vi "App_Training Mode.vi"() -> ()   [LabVIEW 2015, in "Application 1.lvlib"]
uses:
  Application 1.lvlib
  Data Def/App_User Event Data.ctl
  Data Def/App_Subpanel Name.ctl
  Data Def/App_Tips Data.ctl
panel:
  in  "Action":bool
  out "Process":i32(slide) scale=0.0..10.0
  in  "Training Times":i32=10 caption="Numeric" min=1 max=1000 format="%.0f "
  out "Electrocardiography":waveform(dbl)(graph) caption="Waveform Graph"
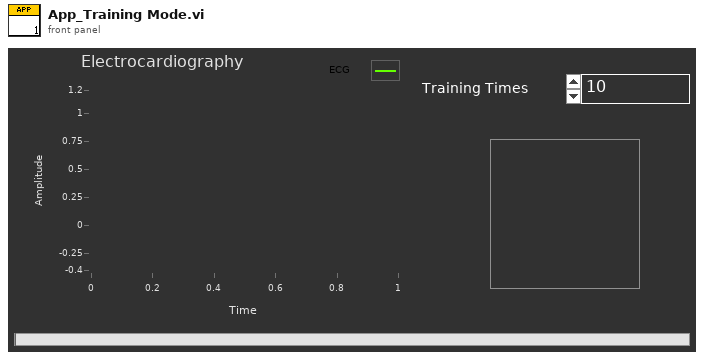
[diagram p1: front panel]
types:
  T1 = typedef "Application 1.lvlib/App_Subpanel Name.ctl" = enum16{"Main", "Menu", "User Registering", "User Setting", "Monitor", "Traning Mode", "Query Data", "Connect Setting"}
  T2 = typedef "Application 1.lvlib/App_User Event Data.ctl" = cluster{"Command":string, "Data":variant}
  T3 = typedef "Application 1.lvlib/App_Tips Data.ctl" = cluster{"Tips":string, "BG Color":u32}
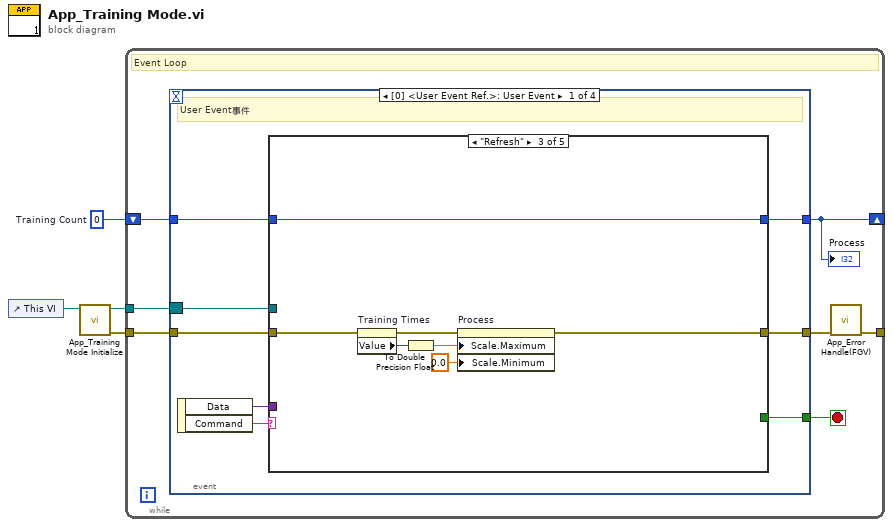
[diagram p0: block diagram]
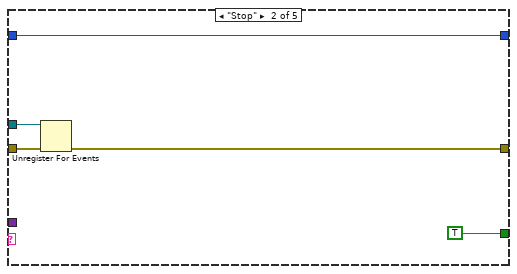
[diagram p3: hidden frame]
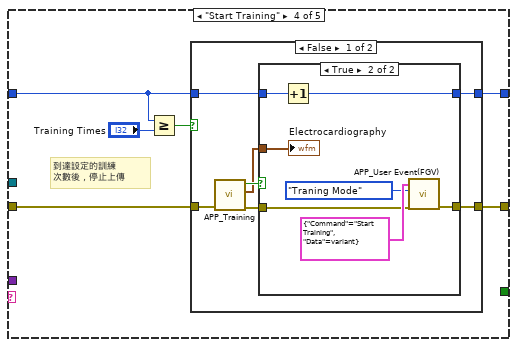
[diagram p4: hidden frame]
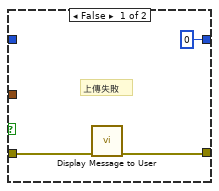
[diagram p5: hidden frame]
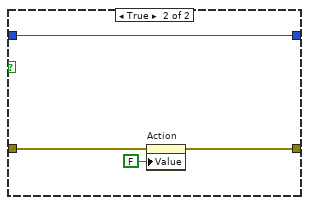
[diagram p6: hidden frame]
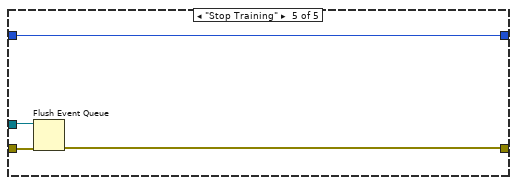
[diagram p7: hidden frame]
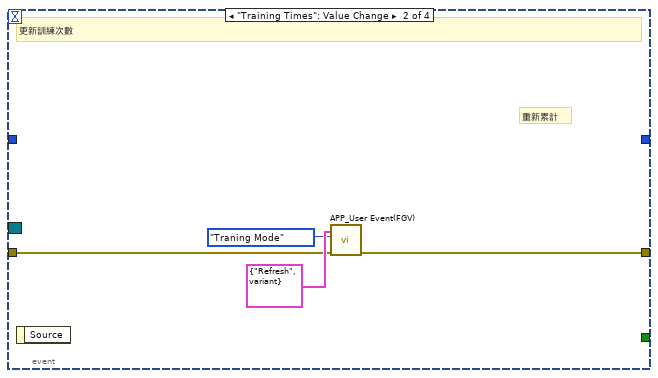
[diagram p8: hidden frame]
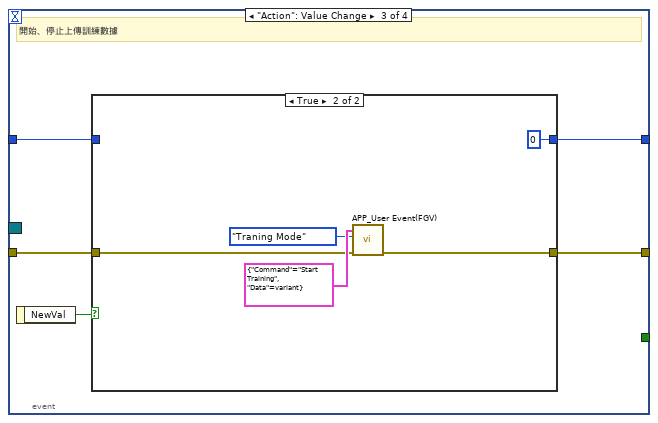
[diagram p9: hidden frame]
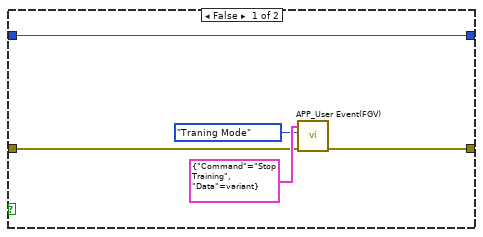
[diagram p10: hidden frame]
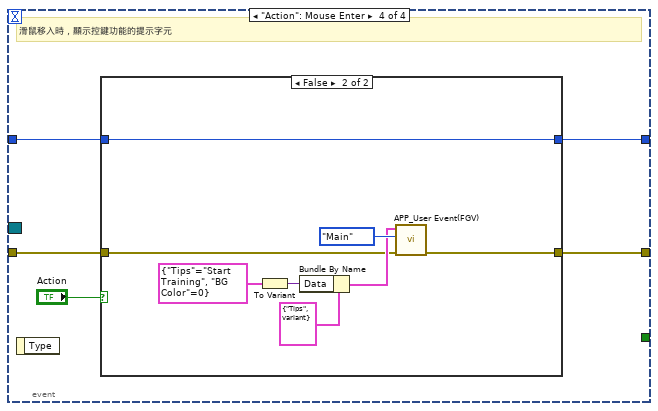
[diagram p11: hidden frame]
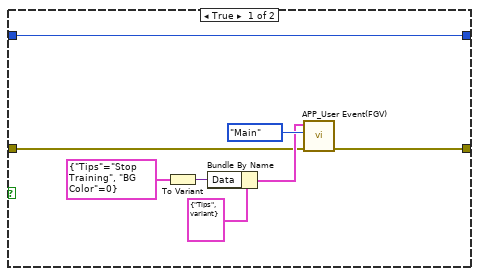
[diagram p12: hidden frame]
diagram:
  w1 = 0  # Training Count
  n1 = control-ref of="This VI"() -> (w4:refnum<vi>)
  n2 = call "App_Training Mode Initialize.vi"("VI Reference"=w4) -> ("error out"=w3:errorcluster, "Event Registration Refnum"=w2:refnum<event-registration>)  [unwired: 9 in]
  n3 = while {
    tunnel: w3 -> [w11]
    tunnel: w2 -> [w10]
    tunnel: [w8] -> _
    shift-right: [w5] -> _
    shift-left: w1 -> [w6]
    stop <- w7 stop-if-true
    # "Event Loop"
    n4 = event shown="[0] <User Event Ref.>: User Event" {
      selector: w10 -> [w15 _ _ _]
      dyn-events: _ -> [_ _ _ _]
      timeout: _ -> [_ _ _ _]
      tunnel: w11 -> [w17 w66 w73 w87]
      tunnel: [w16 w65 w72 w86] -> w9
      tunnel: [w14 _ _ _] -> w7
      tunnel: w6 -> [w13 _ w71 w85]
      tunnel: [w12 _ w70 w84] -> w5
      event User Event {
        # "User Event事件"
        n5 = event-data() -> ("Data"=w18:variant, "Command"=w19:string)  [unwired: 1 in]
        n6 = case shown="\"Refresh\"" w19 {
          tunnel: w18 -> [_ _ _ _ _]
          tunnel: w17 -> [w21 w26 w33 w34 w64]
          tunnel: [w21 w24 w28 w39 w62] -> w16
          tunnel: w15 -> [_ w25 _ _ w63]
          tunnel: [_ TRUE _ _ _] -> w14
          tunnel: w13 -> [w20 w22 w27 w36 w61]
          tunnel: [w20 w22 w27 w38 w61] -> w12
          frame Default {
          }
          frame "Stop" {
            n7 = Unregister For Events(event registration refnum=w25, error in=w26) -> (error out=w24:errorcluster)
          }
          frame "Refresh" {
            n8 = property on="Training Times" class="DigNum (strict)"(error in=w33) -> (error out=w31:errorcluster, "Value"=w32:i32)  [unwired: 1 in, 1 out]
            n9 = To Double Precision Float(number=w32) -> (double precision float=w30:dbl)
            n10 = property on="Process" class="Slide (strict)"(error in=w31, "Scale.Maximum"=w30, "Scale.Minimum"=0.0 ("Scale.Range:Minimum")) -> (error out=w28:errorcluster)  [unwired: 1 in, 1 out]
          }
          frame "Start Training" {
            # "到達設定的訓練\n次數後，停止上傳"
            n11 = Greater Or Equal?(x=w36, y="Training Times") -> (x >= y?=w35:bool)
            n12 = case shown="False" w35 {
              tunnel: w34 -> [w45 w59]
              tunnel: [w46 w57] -> w39
              tunnel: w36 -> [w42 w60]
              tunnel: [w41 w60] -> w38
              frame False {
                n13 = call "APP_Training.vi"("error in"=w45) -> ("error out"=w44:errorcluster, "Data"=w40:waveform(dbl), "OK?"=w43:bool)  [unwired: 8 in]
                n14 = case shown="True" w43 {
                  tunnel: [w47 w54] -> w46
                  tunnel: w44 -> [w48 w53]
                  tunnel: w42 -> [_ w52]
                  tunnel: [0 w51] -> w41
                  tunnel: w40 -> [_ w50]
                  frame False {
                    # "上傳失敗"
                    n15 = call "Display Message to User"("error in (no error)"=w48) -> ("error out"=w47:errorcluster)  [unwired: 9 in, 1 out]
                  }
                  frame True {
                    n16 = Increment(x=w52) -> (x+1=w51:i32)
                    n17 = call "APP_User Event(FGV).vi"("error in"=w53, "Subpanel Name"=App_Subpanel_Name."Traning Mode", "User Event Data"=T2 {"Command"="Start Training", "Data"=variant}) -> ("error out"=w54:errorcluster)  [unwired: 7 in, 1 out]
                    "Electrocardiography" <- w50
                  }
                }
              }
              frame True {
                n18 = property on="Action" class="Bool (strict)"(error in=w59, "Value"=FALSE ("Action")) -> (error out=w57:errorcluster)  [unwired: 1 in, 1 out]
              }
            }
          }
          frame "Stop Training" {
            n19 = Flush Event Queue(0:w63, 3:w64) -> (11:w62:errorcluster)  [unwired: 4 in, 2 out]
          }
        }
      }
      event "Training Times": Value Change {
        # "重新累計"
        # "更新訓練次數"
        n20 = event-data() -> ()  [unwired: 1 in, 1 out]
        n21 = call "APP_User Event(FGV).vi"("error in"=w66, "Subpanel Name"=App_Subpanel_Name."Traning Mode", "User Event Data"=T2 {"Command"="Refresh", "Data"=variant}) -> ("error out"=w65:errorcluster)  [unwired: 7 in, 1 out]
      }
      event "Action": Value Change {
        # "開始、停止上傳訓練數據"
        n22 = event-data() -> ("NewVal"=w69:bool)  [unwired: 1 in]
        n23 = case shown="True" w69 {
          tunnel: w73 -> [w76 w81]
          tunnel: [w75 w80] -> w72
          tunnel: w71 -> [w74 _]
          tunnel: [w74 0 ("Training Count")] -> w70
          frame False {
            n24 = call "APP_User Event(FGV).vi"("error in"=w76, "Subpanel Name"=App_Subpanel_Name."Traning Mode", "User Event Data"=T2 {"Command"="Stop Training", "Data"=variant}) -> ("error out"=w75:errorcluster)  [unwired: 7 in, 1 out]
          }
          frame True {
            n25 = call "APP_User Event(FGV).vi"("error in"=w81, "Subpanel Name"=App_Subpanel_Name."Traning Mode", "User Event Data"=T2 {"Command"="Start Training", "Data"=variant}) -> ("error out"=w80:errorcluster)  [unwired: 7 in, 1 out]
          }
        }
      }
      event "Action": Mouse Enter {
        # "滑鼠移入時，顯示控鍵功能的提示字元"
        n26 = event-data() -> ()  [unwired: 1 in, 1 out]
        n27 = case shown="False" "Action" {
          tunnel: w87 -> [w91 w99]
          tunnel: [w90 w98] -> w86
          tunnel: w85 -> [w89 w97]
          tunnel: [w89 w97] -> w84
          frame True {
            n28 = To Variant(anything=T3 {"Tips"="Stop Training", "BG Color"=0} ("Tips Data")) -> (Variant=w94:variant)
            n29 = Bundle By Name(cluster=T2 {"Command"="Tips", "Data"=variant} ("User Event Data"), "Data"=w94) -> (w93:T2)
            n30 = call "APP_User Event(FGV).vi"("error in"=w91, "Subpanel Name"=App_Subpanel_Name."Main", "User Event Data"=w93) -> ("error out"=w90:errorcluster)  [unwired: 7 in, 1 out]
          }
          frame False {
            n31 = To Variant(anything=T3 {"Tips"="Start Training", "BG Color"=0} ("Tips Data")) -> (Variant=w102:variant)
            n32 = Bundle By Name(cluster=T2 {"Command"="Tips", "Data"=variant} ("User Event Data"), "Data"=w102) -> (w101:T2)
            n33 = call "APP_User Event(FGV).vi"("error in"=w99, "Subpanel Name"=App_Subpanel_Name."Main", "User Event Data"=w101) -> ("error out"=w98:errorcluster)  [unwired: 7 in, 1 out]
          }
        }
      }
    }
    "Process" <- w5
    n34 = call "App_Error Handle(FGV).vi"("error in"=w9) -> ("error out"=w8:errorcluster)  [unwired: 9 in, 1 out]
  }
